vi "GetData.vi"(8 "error in (no error)":errorcluster caption="Fehler (Eingang, kein Fehler)", 10 "Name":string, 11 "Dictionary Eingang":refnum<class "Dictionary.lvclass"> caption="DNL_LabVIEW Object in") -> (0 "error out":errorcluster caption="Fehler (Ausgang)", 2 "Wert":variant, 3 "Dictionary Ausgang":refnum<class "Dictionary.lvclass"> caption="DNL_LabVIEW Object out")   [LabVIEW 2013, in "LvDictionary.lvlib" / "Dictionary.lvclass"]
uses:
  Dictionary.lvclass
  Dictionary.lvclass/Dictionary.ctl
  Properties/GetDict.vi
  <vilib>/Utility/error.llb/Error Cluster From Error Code.vi
  <vilib>/ErrorRing/Error Ring.xnode
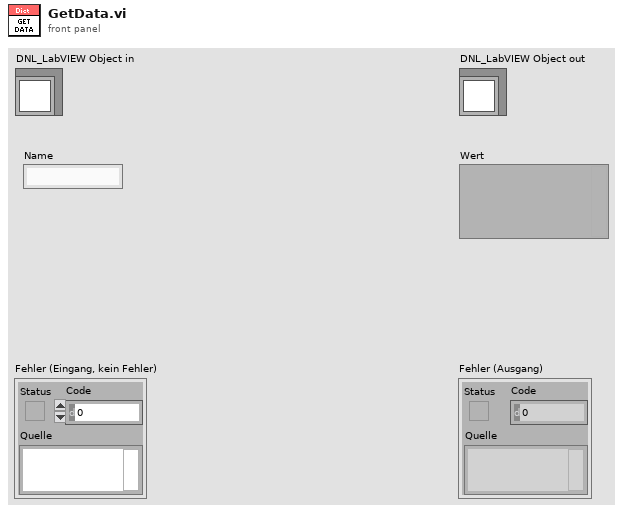
[diagram p1: front panel]
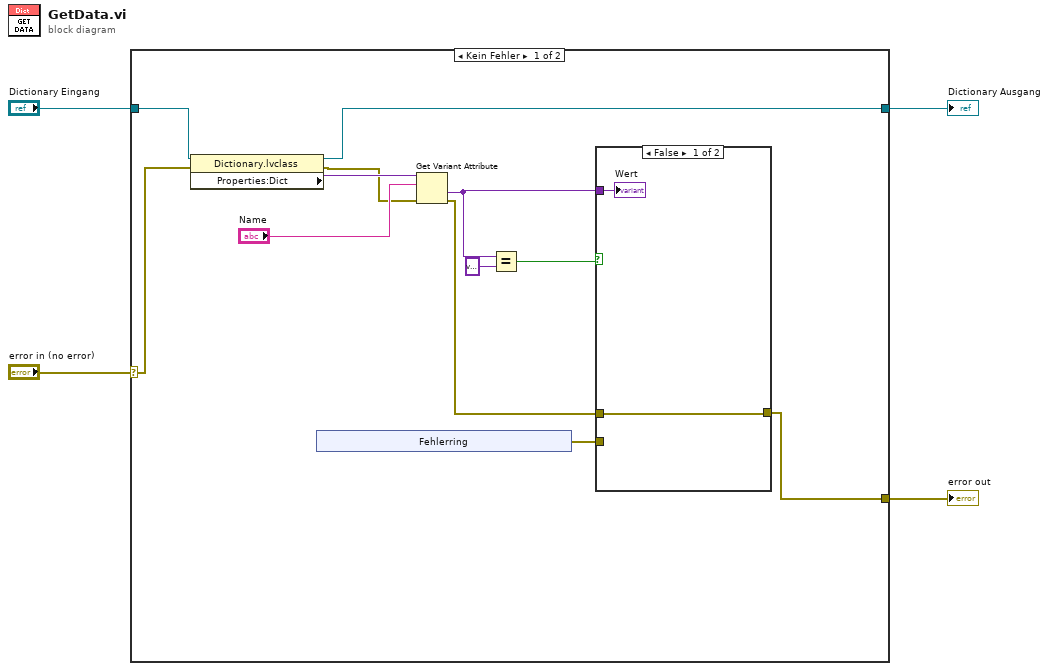
[diagram p0: block diagram]
diagram:
  n1 = case shown="Kein Fehler" "error in (no error)" {
    selector: "error in (no error)" -> [w12 w26]
    tunnel: [w7 w26] -> w3
    tunnel: [w15 w25] -> w1
    tunnel: "Dictionary Eingang" -> [w16 w25]
    frame No Error {
      n2 = property class="Dictionary.lvclass"(reference=w16, error in=w12) -> (reference out=w15:refnum<class "Dictionary.lvclass">, error out=w11:errorcluster, "Properties:Dict"=w14:variant)
      n3 = xnode "Fehlerring"() -> ("Fehler (Ausgang)"=w5:errorcluster)
      n4 = Get Variant Attribute(Variant=w14, name="Name", error in=w11) -> (value=w6:variant, error out=w8:errorcluster)  [unwired: 1 in, 2 out]
      n5 = Equal?(x=w6, y=variant) -> (x = y?=w9:bool)
      n6 = case shown="False" w9 {
        tunnel: w8 -> [w23 _]
        tunnel: [w23 w24] -> w7
        tunnel: w6 -> [w22 _]
        tunnel: w5 -> [_ w24]
        frame False {
          "Wert" <- w22
        }
        frame True {
        }
      }
    }
    frame Error {
    }
  }
  "error out" <- w3
  "Dictionary Ausgang" <- w1
